vi "Sub_KDELTA_delFix.vi"(9 "Pin-Location":i32, 10 "Pre-Pin Matrix":dbl[][](array[numeric])) -> (3 "K12":dbl[][](array[numeric]))   [LabVIEW 2019]
uses:
  <vilib>/Analysis/Matrix/Numeric/Conversions/Matrix To Array - RM.vi
  <vilib>/Analysis/Matrix/NI_Matrix.lvlib
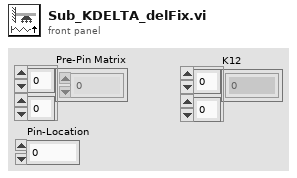
[diagram p1: front panel]
types:
  T1 = typedef "NI_Matrix.lvlib/RealMatrix.ctl" = dbl[][]
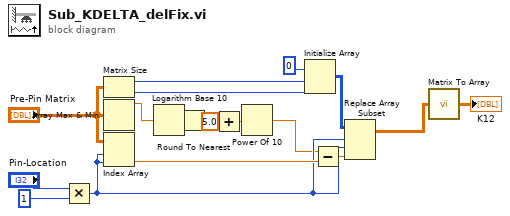
[diagram p0: block diagram]
diagram:
  n1 = Multiply(x="Pin-Location", y=1) -> (x*y=w8:i32)
  n2 = Matrix Size(0:"Pre-Pin Matrix") -> (1:w13:i32, 2:w14:i32)
  n3 = Array Max & Min(array="Pre-Pin Matrix") -> (max value=w2:dbl)  [unwired: 3 out]
  n4 = Index Array(array="Pre-Pin Matrix", index (row)=w8, index (col)=w8) -> (element=w10:dbl)
  n5 = Logarithm Base 10(1:w2) -> (0:w6:dbl)
  n6 = Round To Nearest(number=w6) -> (nearest integer value=w5:dbl)
  n7 = Add(x=w5, y=5.0) -> (x+y=w3:dbl)
  n8 = Power Of 10(x=w3) -> (10^x=w1:dbl)
  n9 = Initialize Array(0, w13, w14) -> (w9:i32[][])
  n10 = Subtract(x=w1, y=w10) -> (x-y=w11:dbl)
  n11 = Replace Array Subset(array=w9, new element=w11, index (row)=w8, index (col)=w8) -> (w17:T1)
  n12 = call-poly <vilib>:"Matrix To Array.vi"("Real Matrix"=w17) -> ("Real 2D Array"=→"K12":dbl[][])
